vi "Read App Item_.vi"(8 "error in (no error)":errorcluster, 11 "MenuActivationMsg in":refnum<class "MenuActivationMsg.lvclass">) -> (0 "error out":errorcluster, 2 "App Item?":bool, 3 "MenuActivationMsg out":refnum<class "MenuActivationMsg.lvclass">)   [LabVIEW 2020, in "ActorEvents.lvlib" / "MenuActivationMsg.lvclass"]
uses:
  <vilib>/gpm_packages/@cs/mva-viewable/Source/ActorEvents/IEventAggregator Messages/Menu Activation Msg/MenuActivationMsg.lvclass
  <vilib>/gpm_packages/@cs/mva-viewable/Source/ActorEvents/IEventAggregator Messages/Menu Activation Msg/MenuActivationMsg.lvclass/MenuActivationMsg.ctl
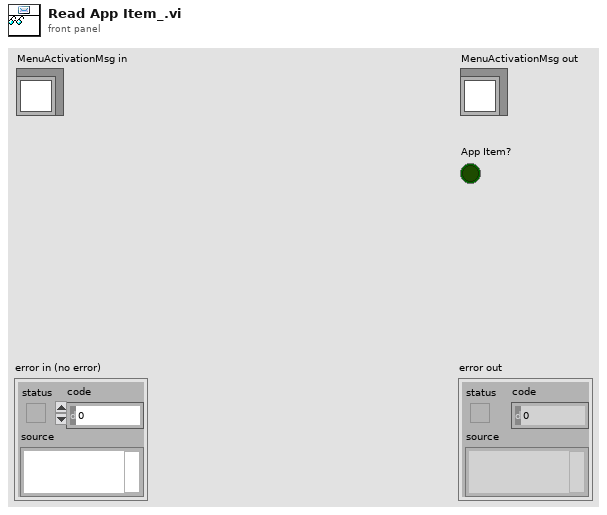
[diagram p1: front panel]
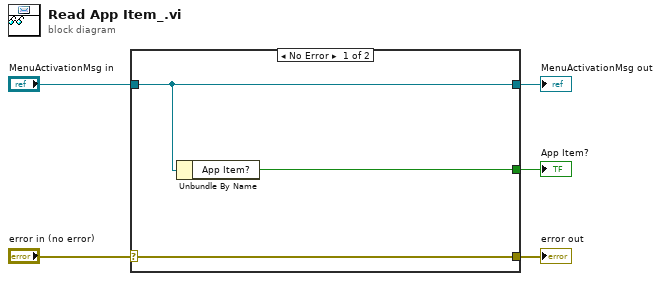
[diagram p0: block diagram]
diagram:
  n1 = case shown="No Error" "error in (no error)" {
    selector: "error in (no error)" -> [w8 w9]
    tunnel: [w8 w9] -> w4
    tunnel: [w7 w10] -> w2
    tunnel: "MenuActivationMsg in" -> [w7 w10]
    tunnel: [w6 _] -> w1
    frame No Error {
      n2 = Unbundle By Name(w7) -> ("App Item?"=w6:bool)
    }
    frame Error {
    }
  }
  "error out" <- w4
  "MenuActivationMsg out" <- w2
  "App Item?" <- w1
